vi "3.2.0 Kalman Update Matrix F.vi"(0 "3.2.0 Kalman dt":dbl=0.05, 1 "State Vector X":T1) -> (3 "Update Matrix F":T2 format="%_6e")   [LabVIEW 2010]
uses:
  4-High Neurons/4.2/4.2.0 Kalman State.ctl
  <vilib>/Analysis/Matrix/Datatypes/RealMatrix.ctl
  <vilib>/Analysis/7linalg.llb/Create Special Real Matrix.vi
  <vilib>/Analysis/Matrix/Numeric/Conversions/Array To Matrix - RA.vi
  3.0-Global.vi
  <vilib>/Analysis/baseanly.llb/Real A x B.vi
  <vilib>/Analysis/NI_AALPro.lvlib
  <vilib>/Analysis/Matrix/NI_Matrix.lvlib
  <vilib>/Analysis/NI_AALBase.lvlib
panel:
  out "delta theta":dbl
  out "Arc Length Traveled by Center":dbl
  out "Ratio of Center to Front":dbl
  out "Arc Length Traveled By Front Wheel":dbl
  out "atan2(y,x)":dbl
  out "New state would be":T1
  out "A x B":T2
  out "Front Wheel Radius":dbl
  out "Alternate formulation":dbl
  out "Center Radius":dbl
  out "Tan^2(w)*V^2/l^2":dbl
  out "W/Wd":dbl
  out "V/V":dbl
  out "O/V":dbl
  out "Y/V":dbl
  out "X/V":dbl
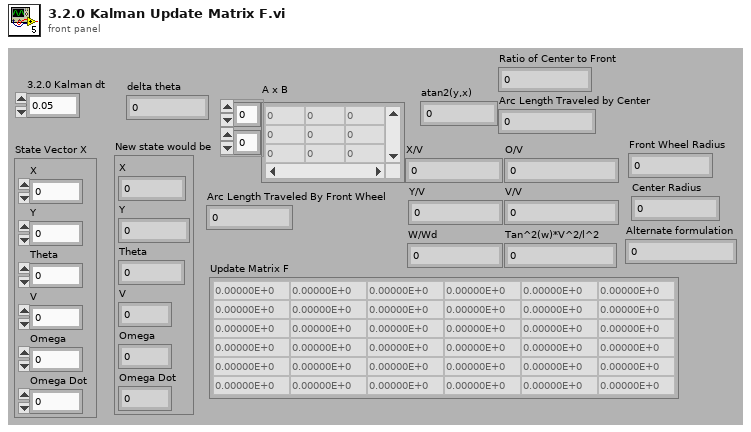
[diagram p1: front panel]
types:
  T1 = typedef "4.2.0 Kalman State.ctl" = cluster{"X":dbl, "Y":dbl, "Theta":dbl, "V":dbl, "Omega":dbl, "Omega Dot":dbl}
  T2 = typedef "NI_Matrix.lvlib/RealMatrix.ctl" = dbl[][]
  T3 = enum32{"Identity", "Diagonal", "Toepliz", "Vandermonde", "Companion"}
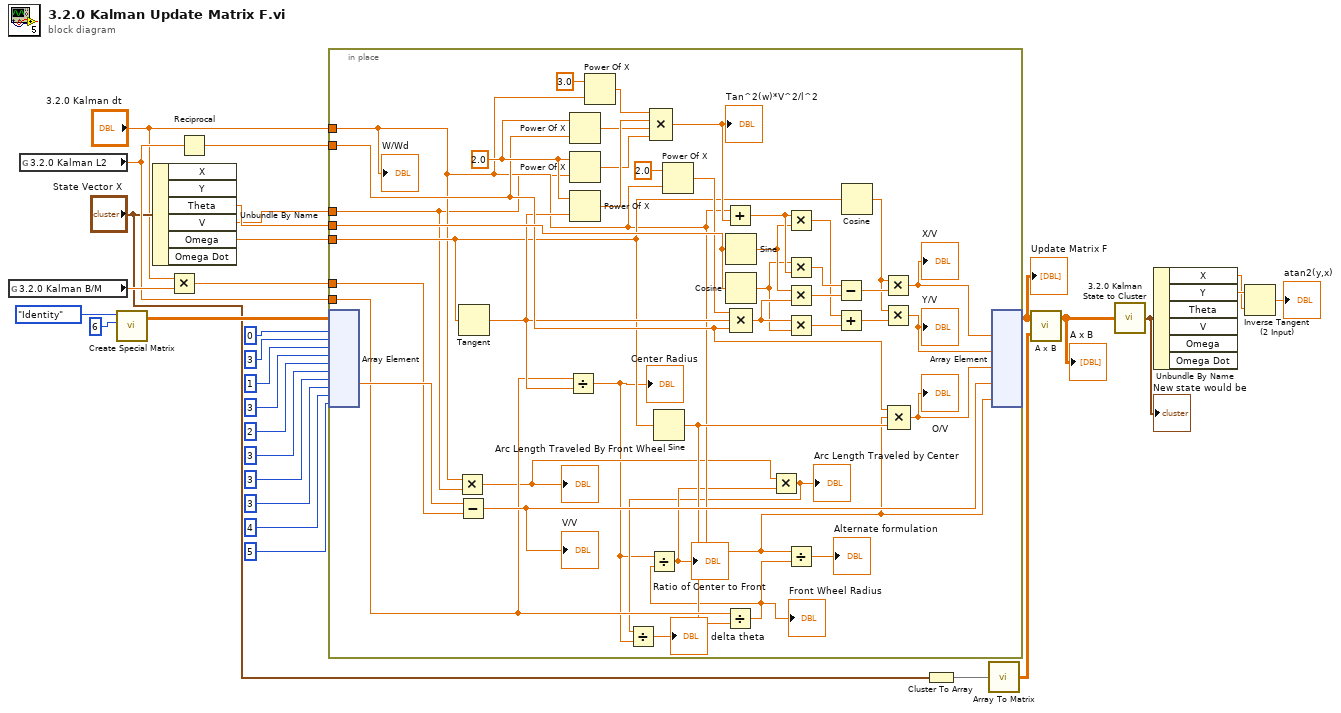
[diagram p0: block diagram]
diagram:
  n1 = global read "3.0-Global.vi" "3.2.0 Kalman B/M"() -> (w13:dbl)
  n2 = global read "3.0-Global.vi" "3.2.0 Kalman L2"() -> (w11:dbl)
  n3 = call-poly <vilib>:"Create Special Matrix.vi"("matrix type"=T3."Identity", "matrix size"=6) -> ("Special Matrix"=w16:T2)  [unwired: 3 in, 1 out]
  n4 = Unbundle By Name("State Vector X") -> ("Theta"=w30:dbl, "V"=w28:dbl, "Omega"=w29:dbl)  [unwired: 3 out]
  n5 = Multiply(x="3.2.0 Kalman dt", y=w13) -> (x*y=w12:dbl)
  n6 = Reciprocal(x=w11) -> (1/x=w19:dbl)
  n7 = in-place {
    in-place-border: w30 -> [w63]
    in-place-border: "3.2.0 Kalman dt" -> [w38]
    in-place-border: w29 -> [w41]
    in-place-border: w19 -> [w51]
    in-place-border: w28 -> [w37]
    in-place-border: w12 -> [w47]
    in-place-border: w11 -> [w40]
    w70 = 2.0 ("y")
    n8 = in-place-array #1(w16, 0, 3, 1, 3, 2, 3, 3, 3, 4, 5) -> (w49:dbl)  [unwired: 4 out]
    n9 = Multiply(x=w38, y=w37) -> (x*y=w34:dbl)
    "Arc Length Traveled By Front Wheel" <- w34
    n10 = Subtract(x=w49, y=w47) -> (x-y=w48:dbl)
    "V/V" <- w48
    n11 = Tangent(1:w41) -> (0:w46:dbl)
    n12 = Divide(x=w40, y=w46) -> (x/y=w32:dbl)
    "Center Radius" <- w32
    n13 = Power Of X(1:w51, 2:w70) -> (0:w67:dbl)
    n14 = Power Of X(1:w37, 2:w70) -> (0:w66:dbl)
    n15 = Power Of X(1:w46, 2:w70) -> (0:w68:dbl)
    n16 = Power Of X(1:w38, 2:3.0 ("y")) -> (0:w69:dbl)
    n17 = Compound Arithmetic op=MULTIPLY(w69, w68, w67, w66) -> (w65:dbl)
    "Tan^2(w)*V^2/l^2" <- w65
    n18 = Sine(x=w41) -> (sin(x)=w39:dbl)
    n19 = Power Of X(1:w38, 2:2.0 ("y")) -> (0:w61:dbl)
    n20 = Add(x=w38, y=w65) -> (x+y=w58:dbl)
    n21 = Divide(x=w40, y=w39) -> (x/y=w36:dbl)
    "Front Wheel Radius" <- w36
    n22 = Divide(x=w32, y=w36) -> (x/y=w35:dbl)
    "Ratio of Center to Front" <- w35
    n23 = Sine(x=w63) -> (sin(x)=w57:dbl)
    n24 = Cosine(x=w63) -> (cos(x)=w55:dbl)
    n25 = Compound Arithmetic op=MULTIPLY(w61, w46, w51) -> (w56:dbl)
    n26 = Multiply(x=w34, y=w35) -> (x*y=w33:dbl)
    "Arc Length Traveled by Center" <- w33
    n27 = Divide(x=w33, y=w32) -> (x/y=→"delta theta":dbl)
    n28 = Multiply(x=w58, y=w57) -> (x*y=w54:dbl)
    n29 = Multiply(x=w55, y=w58) -> (x*y=w64:dbl)
    n30 = Multiply(x=w57, y=w56) -> (x*y=w59:dbl)
    n31 = Multiply(x=w56, y=w55) -> (x*y=w53:dbl)
    n32 = Divide(x=w38, y=w36) -> (x/y=→"Alternate formulation":dbl)
    n33 = Subtract(x=w64, y=w59) -> (x-y=w60:dbl)
    n34 = Add(x=w54, y=w53) -> (x+y=w52:dbl)
    n35 = Cosine(x=w41) -> (cos(x)=w42:dbl)
    n36 = Multiply(x=w42, y=w60) -> (x*y=w44:dbl)
    "X/V" <- w44
    n37 = Multiply(x=w42, y=w52) -> (x*y=w43:dbl)
    "Y/V" <- w43
    n38 = Compound Arithmetic op=MULTIPLY(w51, w38, w39) -> (w50:dbl)
    "O/V" <- w50
    n39 = in-place-array #1(w44, w43, w50, w48, w38) -> (w7:T2)  [unwired: 10 out]
    "W/Wd" <- w38
  }
  "Update Matrix F" <- w7
  n40 = Cluster To Array(cluster="State Vector X") -> (array=w9:dbl[])
  n41 = call-poly <vilib>:"Array To Matrix.vi"("Real 1D Array"=w9) -> ("Real Matrix (Column Vector)"=w8:T2)
  n42 = call-poly <vilib>:"A x B.vi"("B"=w8, "A"=w7) -> ("A x B"=w6:T2)  [unwired: 1 out]
  "A x B" <- w6
  n43 = call "3.2.0 Kalman State to Cluster.vi"("State Variable X 3"=w6) -> ("State Vector X"=w5:T1)
  "New state would be" <- w5
  n44 = Unbundle By Name(w5) -> ("X"=w3:dbl, "Y"=w4:dbl)  [unwired: 4 out]
  n45 = Inverse Tangent (2 Input)(1:w3, 2:w4) -> (0:→"atan2(y,x)":dbl)
